vi "Sys config window-Update general setup.vi"(8 "error in (no error)":errorcluster, 10 "Calibration settings":T1, 11 "General Setup":T2={"Microscope ID"="003", "Microscope Type"="AOLM", "Revision Number"="1.0.0.0", "Advanced Imaging"=FALSE, "Error Logging"=FALSE, "Performance Monitoring"=FALSE, "Max Allowed Trial Length"=60.0, "Initial Scan Resolution"=512.0, "Initial Acceptance Angle"=5.0, "Initial Laser Wavelength"=900.0, "Initial Dwell Time"=900.0}) -> (0 "error out":errorcluster)   [LabVIEW 2020]
uses:
  Typedefs/General Setup.ctl
  Configuration code/Typedefs/Pockels Calibration settings cluster.ctl
  Typedefs/fgv_actions.ctl
  Global Variables/General Globals.vi
  Configuration code/Calibration/Globals/gl_Calibration globals.vi
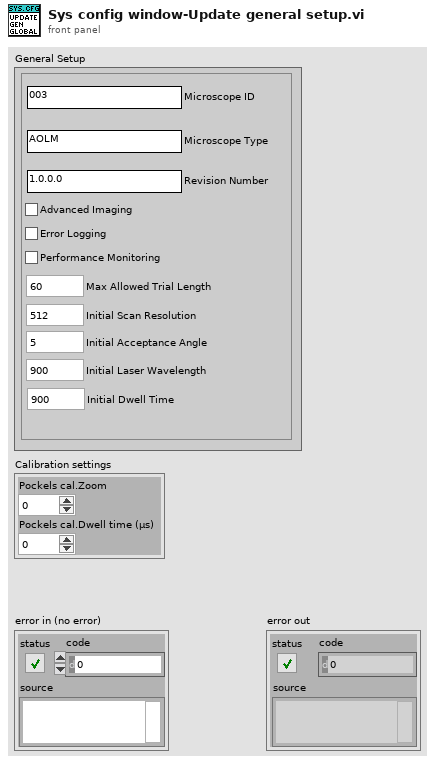
[diagram p1: front panel]
types:
  T1 = typedef "Pockels Calibration settings cluster.ctl" = cluster{"Pockels cal.Zoom":u8, "Pockels cal.Dwell time (µs)":dbl}
  T2 = typedef "General Setup.ctl" = cluster{"Microscope ID":string, "Microscope Type":string, "Revision Number":string, "Advanced Imaging":bool, "Error Logging":bool, "Performance Monitoring":bool, "Max Allowed Trial Length":dbl, "Initial Scan Resolution":dbl, "Initial Acceptance Angle":dbl, "Initial Laser Wavelength":dbl, "Initial Dwell Time":dbl}
  T3 = typedef "fgv_actions.ctl" = enum16{"Get", "Set"}
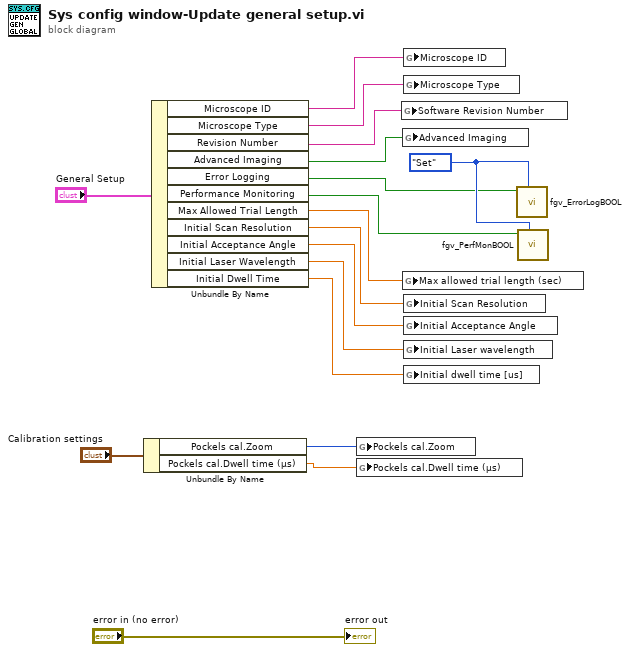
[diagram p0: block diagram]
diagram:
  w12 = fgv_actions."Set" ("FGV Actions")
  n1 = Unbundle By Name("Calibration settings") -> ("Pockels cal.Zoom"=w3:u8, "Pockels cal.Dwell time (µs)"=w2:dbl)
  n2 = Unbundle By Name("General Setup") -> ("Microscope ID"=w16:string, "Microscope Type"=w15:string, "Revision Number"=w14:string, "Advanced Imaging"=w13:bool, "Error Logging"=w11:bool, "Performance Monitoring"=w10:bool, "Max Allowed Trial Length"=w9:dbl, "Initial Scan Resolution"=w8:dbl, "Initial Acceptance Angle"=w7:dbl, "Initial Laser Wavelength"=w6:dbl, "Initial Dwell Time"=w5:dbl)
  n3 = global write "gl_Calibration globals.vi" "Pockels cal.Zoom"(w3) -> ()
  n4 = global write "gl_Calibration globals.vi" "Pockels cal.Dwell time (µs)"(w2) -> ()
  n5 = global write "General Globals.vi" "Software Revision Number"(w14) -> ()
  n6 = global write "General Globals.vi" "Advanced Imaging"(w13) -> ()
  n7 = global write "General Globals.vi" "Max allowed trial length (sec)"(w9) -> ()
  n8 = global write "General Globals.vi" "Microscope ID"(w16) -> ()
  n9 = global write "General Globals.vi" "Microscope Type"(w15) -> ()
  n10 = global write "General Globals.vi" "Initial Scan Resolution"(w8) -> ()
  n11 = global write "General Globals.vi" "Initial Acceptance Angle"(w7) -> ()
  n12 = global write "General Globals.vi" "Initial Laser wavelength"(w6) -> ()
  n13 = global write "General Globals.vi" "Initial dwell time [us]"(w5) -> ()
  n14 = call "fgv_ErrorLogBOOL.vi"("FGV Actions"=w12, "Error Logging ON [IN] ?"=w11) -> ()  [unwired: 8 in, 2 out]
  n15 = call "fgv_PerfMonBOOL.vi"("FGV Actions"=w12, "Perf Mon [IN]"=w10) -> ()  [unwired: 8 in, 2 out]
  "error out" <- "error in (no error)"
